vi "Configure Standard Waveform.vi"(4 "Unit (0: Vpp)":u16(ring) items=["Vpp", "Vrms", "dB"], 6 "DC Offset (0.00 V)":dbl, 7 "Frequency (1000 Hz)":dbl=1000.0, 8 "error in (no error)":errorcluster, 9 "Amplitude (1)":dbl=1.0, 10 "Waveform Function (1: Sine)":u16(ring)=1 items=["DC", "Sine", "Square", "Triangle", "Ramp", "Pulse", "Noise", "Sinc", "Negative Ramp", "Exponential Rise", "Exponential Fall", "Cardiac"], 11 "VISA resource name":refnum<visa-resource-name>) -> (0 "error out":errorcluster, 3 "VISA resource name out":refnum<visa-resource-name>)   [LabVIEW 2012, in "Agilent 33XXX Series.lvlib"]
doc: "Selects the waveform shape, frequency, amplitude, offset, and phase for a standard waveform."
uses:
  Agilent 33XXX Series.lvlib
panel:
  out "resulting string":string
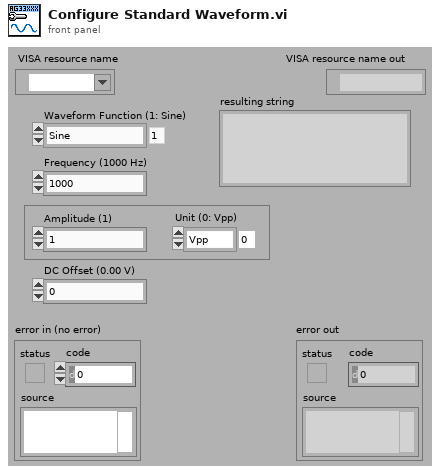
[diagram p1: front panel]
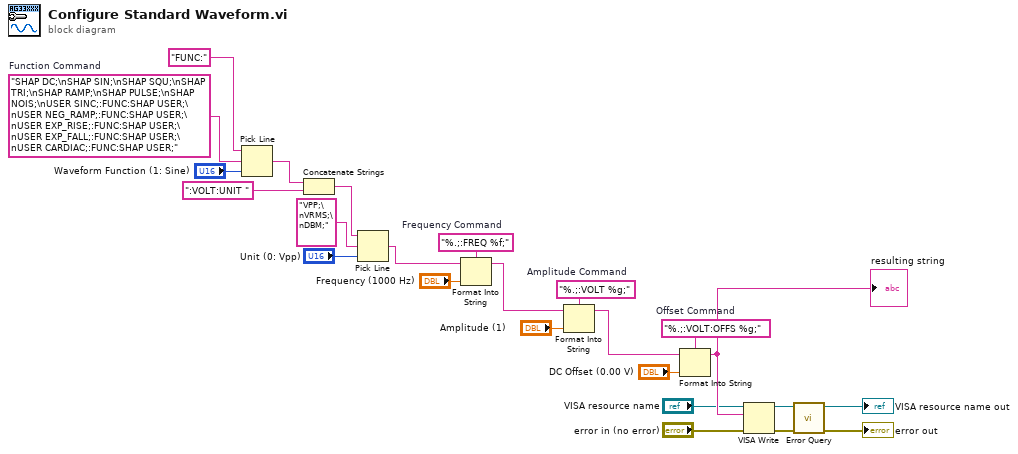
[diagram p0: block diagram]
diagram:
  w19 = "%.;:VOLT:OFFS %g;"  # Offset Command
  w20 = "%.;:VOLT %g;"  # Amplitude Command
  w21 = "%.;:FREQ %f;"  # Frequency Command
  w22 = "SHAP DC;\nSHAP SIN;\nSHAP SQU;\nSHAP TRI;\nSHAP RAMP;\nSHAP PULSE;\nSHAP NOIS;\nUSER SINC;:FUNC:SHAP USER;\nUSER NEG_RAMP;:FUNC:SHAP USER;\nUSER EXP_RISE;:FUNC:SHAP USER;\nUSER EXP_FALL;:FUNC:SHAP USER;\nUSER CARDIAC;:FUNC:SHAP USER;"  # Function Command
  n1 = Pick Line(string ("")="FUNC:", multi-line string=w22, line index="Waveform Function (1: Sine)") -> (output string=w9:string)
  n2 = Concatenate Strings(w9, ":VOLT:UNIT ") -> (w10:string)
  n3 = Pick Line(string ("")=w10, multi-line string="VPP;\nVRMS;\nDBM;", line index="Unit (0: Vpp)") -> (output string=w8:string)
  n4 = Format Into String(format string=w21, initial string=w8, "Frequency (1000 Hz)") -> (resulting string=w14:string)  [unwired: 1 in, 1 out]
  n5 = Format Into String(format string=w20, initial string=w14, "Amplitude (1)") -> (resulting string=w15:string)  [unwired: 1 in, 1 out]
  n6 = Format Into String(format string=w19, initial string=w15, "DC Offset (0.00 V)") -> (resulting string=w6:string)  [unwired: 1 in, 1 out]
  "resulting string" <- w6
  n7 = VISA Write(VISA resource name="VISA resource name", write buffer=w6, error in (no error)="error in (no error)") -> (VISA resource name out=w24:refnum<visa-resource-name>, error out=w23:errorcluster)  [unwired: 1 out]
  n8 = call "Error Query.vi"("error in (no error)"=w23, "VISA resource name"=w24) -> ("error out"=→"error out":errorcluster, "VISA resource name out"=→"VISA resource name out":refnum<visa-resource-name>)  [unwired: 6 in, 2 out]
